vi "UPRESULT.vi"(0 "DEVICE_ID":string, 5 "USER_ID":string, 7 "CODE_ID":string, 9 "RESULT_VALUE":string, 11 "错误输入":errorcluster) -> (15 "error out":errorcluster)   [LabVIEW 2020]
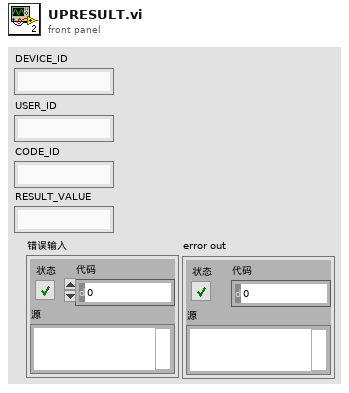
[diagram p1: front panel]
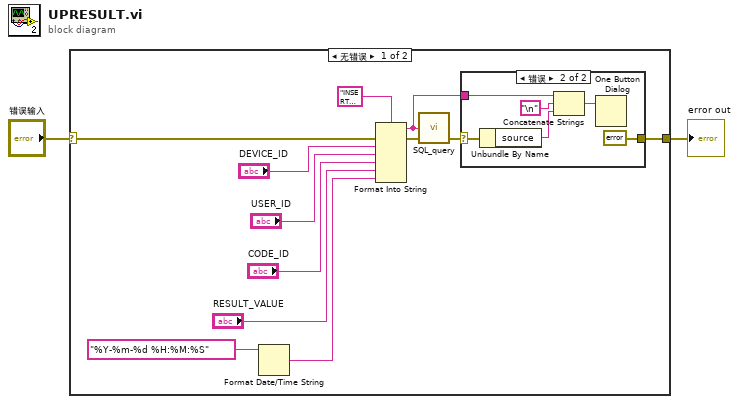
[diagram p0: block diagram]
diagram:
  n1 = case shown="无错误" "错误输入" {
    selector: "错误输入" -> [w6 w22]
    tunnel: [w4 w22] -> w1
    frame No Error {
      n2 = Format Date/Time String(time format string (%c)="%Y-%m-%d %H:%M:%S" ("时间格式字符串(%c)")) -> (date/time string=w13:string)  [unwired: 2 in]
      n3 = Format Into String(format string="INSERT INTO [dbo].[Result] ( [DEVICE_ID], [USER_ID], [CODE_ID], [RESULT_VALUE], [RESULT_TIME] ) \nVALUES\n\t( %s, %s, %s, N'%s', '%s' ) ", error in=w6, "DEVICE_ID", "USER_ID", "CODE_ID", "RESULT_VALUE", w13) -> (resulting string=w3:string, error out=w14:errorcluster)  [unwired: 1 in]
      n4 = call "SQL_query.vi"("error in (no error)"=w14, "SQL query"=w3) -> ("error out"=w5:errorcluster)  [unwired: 1 in, 2 out]
      n5 = case shown="错误" w5 {
        selector: w5 -> [w15 w19]
        tunnel: [w15 errorcluster {"status"=FALSE, "code"=0, "source"=""} ("error IO")] -> w4
        tunnel: w3 -> [_ w21]
        frame No Error {
        }
        frame Error {
          n6 = Unbundle By Name(w19) -> ("source"=w18:string)
          n7 = Concatenate Strings(w21, "\n", w18) -> (w17:string)
          n8 = One Button Dialog(message=w17) -> ()  [unwired: 1 in, 1 out]
        }
      }
    }
    frame Error {
    }
  }
  "error out" <- w1
